vi "5_1_2.vi"() -> ()   [LabVIEW 2025, in "2022.lvlib"]
uses:
  2022.lvlib
  <vilib>/Utility/miscctls.llb/LVMapReplaceAction.ctl
panel:
  in  "Solution":bool
  out "string":string
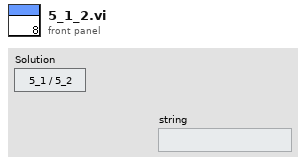
[diagram p1: front panel]
types:
  T1 = cluster{"Crane Stock":string, "Procedure":string}
  T2 = typedef "LVMapReplaceAction.ctl" = enum32{"Modify Entry only if found", "Add or Modify Entry", "Delete Entry"}
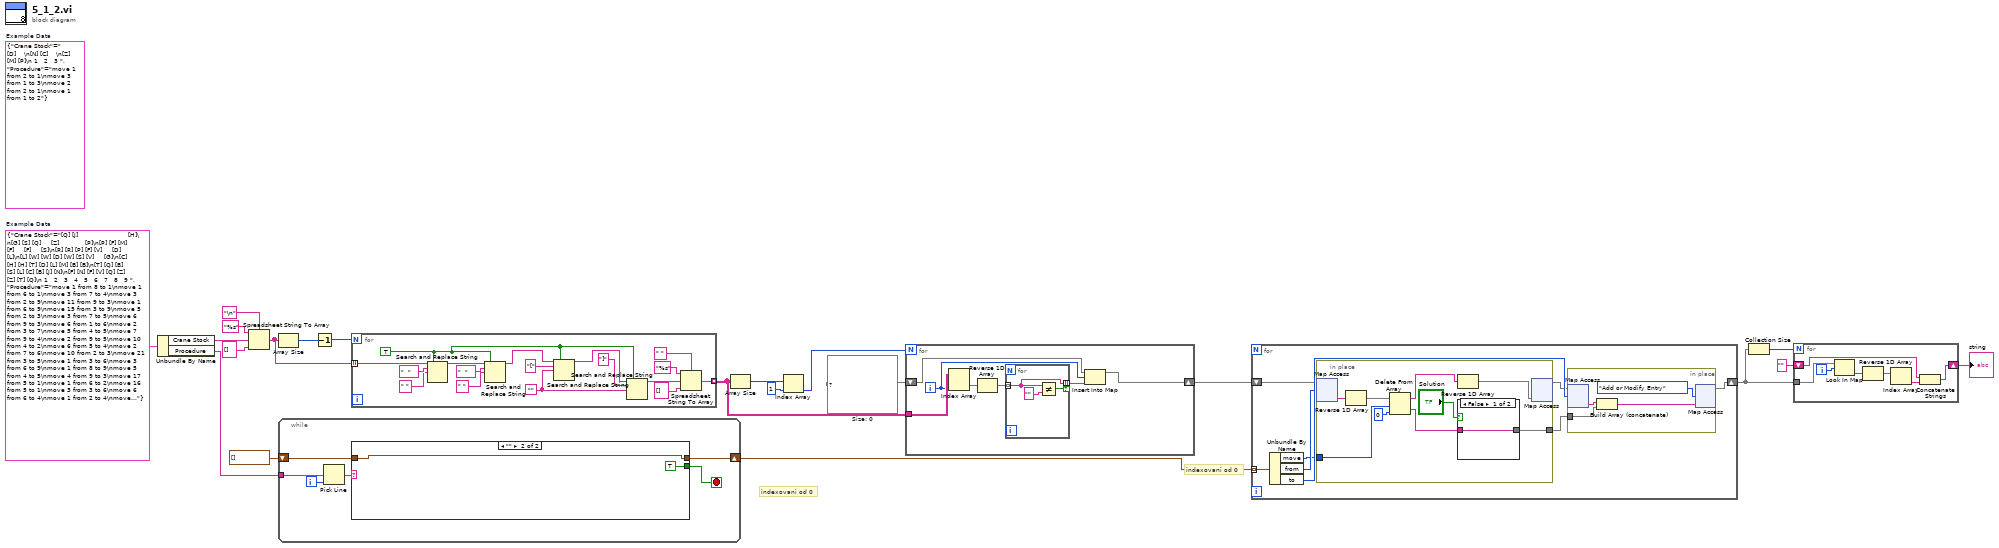
[diagram p0: block diagram]
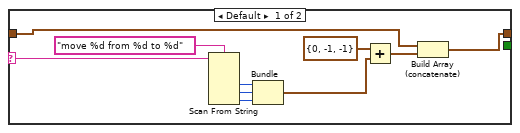
[diagram p2: hidden frame]
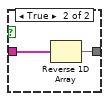
[diagram p3: hidden frame]
diagram:
  (unwired) T1 {"Crane Stock"="   [D]    \n[N] [C]    \n[Z] [M] [P]\n 1   2   3 ", "Procedure"="move 1 from 2 to 1\nmove 3 from 1 to 3\nmove 2 from 2 to 1\nmove 1 from 1 to 2"}  # Example Data
  w12 = map{i32, string[]} {}  # Size: 0
  w1 = T1 {"Crane Stock"="[Q] [J]                         [H]\n[G] [S] [Q]     [Z]             [P]\n[P] [F] [M]     [F]     [F]     [S]\n[R] [R] [P] [F] [V]     [D]     [L]\n[L] [W] [W] [D] [W] [S] [V]     [G]\n[C] [H] [H] [T] [D] [L] [M] [B] [B]\n[T] [Q] [B] [S] [L] [C] [B] [J] [N]\n[F] [N] [F] [V] [Q] [Z] [Z] [T] [Q]\n 1   2   3   4   5   6   7   8   9 ", "Procedure"="move 1 from 8 to 1\nmove 1 from 6 to 1\nmove 3 from 7 to 4\nmove 3 from 2 to 9\nmove 11 from 9 to 3\nmove 1 from 6 to 9\nmove 15 from 3 to 9\nmove 5 from 2 to 3\nmove 3 from 7 to 5\nmove 6 from 9 to 3\nmove 6 from 1 to 6\nmove 2 from 3 to 7\nmove 5 from 4 to 5\nmove 7 from 9 to 4\nmove 2 from 9 to 5\nmove 10 from 4 to 2\nmove 6 from 5 to 4\nmove 2 from 7 to 6\nmove 10 from 2 to 3\nmove 21 from 3 to 5\nmove 1 from 3 to 6\nmove 3 from 6 to 9\nmove 1 from 8 to 9\nmove 5 from 4 to 5\nmove 4 from 9 to 3\nmove 17 from 5 to 1\nmove 1 from 6 to 2\nmove 16 from 5 to 1\nmove 3 from 3 to 6\nmove 6 from 6 to 4\nmove 1 from 2 to 4\nmove 4 from 1 to 2\nmove 2 from 6 to 2\nmove 28 from 1 to 3\nmove 1 from 9 to 7\nmove 1 from 8 to 7\nmove 1 from 5 to 4\nmove 1 from 2 to 6\nmove 1 from 3 to 1\nmove 3 from 2 to 5\nmove 1 from 6 to 3\nmove 4 from 4 to 7\nmove 5 from 5 to 2\nmove 1 from 5 to 6\nmove 6 from 1 to 3\nmove 1 from 6 to 2\nmove 26 from 3 to 6\nmove 2 from 7 to 9\nmove 4 from 7 to 3\nmove 19 from 6 to 3\nmove 6 from 2 to 4\nmove 5 from 3 to 2\nmove 1 from 9 to 7\nmove 26 from 3 to 8\nmove 6 from 4 to 3\nmove 1 from 3 to 8\nmove 1 from 6 to 7\nmove 6 from 3 to 6\nmove 6 from 6 to 4\nmove 1 from 9 to 2\nmove 2 from 4 to 9\nmove 22 from 8 to 2\nmove 2 from 6 to 5\nmove 1 from 9 to 1\nmove 1 from 6 to 5\nmove 1 from 7 to 5\nmove 3 from 6 to 7\nmove 2 from 6 to 1\nmove 1 from 1 to 5\nmove 3 from 5 to 9\nmove 4 from 8 to 4\nmove 2 from 1 to 4\nmove 18 from 2 to 1\nmove 2 from 7 to 8\nmove 3 from 9 to 5\nmove 8 from 1 to 9\nmove 5 from 9 to 3\nmove 1 from 9 to 8\nmove 2 from 9 to 4\nmove 2 from 7 to 8\nmove 5 from 5 to 7\nmove 1 from 9 to 3\nmove 4 from 8 to 4\nmove 1 from 7 to 8\nmove 4 from 4 to 3\nmove 2 from 8 to 3\nmove 1 from 8 to 9\nmove 2 from 1 to 8\nmove 3 from 4 to 5\nmove 1 from 8 to 4\nmove 1 from 9 to 3\nmove 1 from 8 to 5\nmove 8 from 1 to 8\nmove 11 from 2 to 9\nmove 12 from 3 to 5\nmove 1 from 3 to 9\nmove 1 from 8 to 5\nmove 11 from 9 to 3\nmove 4 from 5 to 9\nmove 3 from 8 to 7\nmove 3 from 7 to 8\nmove 1 from 5 to 8\nmove 7 from 4 to 3\nmove 1 from 4 to 5\nmove 1 from 2 to 8\nmove 3 from 7 to 6\nmove 3 from 4 to 8\nmove 1 from 7 to 9\nmove 2 from 4 to 7\nmove 5 from 8 to 1\nmove 3 from 6 to 5\nmove 2 from 4 to 2\nmove 1 from 9 to 4\nmove 1 from 8 to 6\nmove 1 from 2 to 9\nmove 1 from 8 to 5\nmove 3 from 8 to 4\nmove 3 from 4 to 2\nmove 4 from 3 to 9\nmove 17 from 5 to 9\nmove 9 from 9 to 6\nmove 1 from 9 to 3\nmove 5 from 6 to 3\nmove 3 from 6 to 3\nmove 8 from 9 to 5\nmove 2 from 8 to 5\nmove 1 from 4 to 8\nmove 1 from 5 to 3\nmove 1 from 8 to 5\nmove 3 from 2 to 6\nmove 3 from 1 to 4\nmove 7 from 5 to 1\nmove 1 from 2 to 6\nmove 13 from 3 to 6\nmove 2 from 7 to 8\nmove 13 from 6 to 5\nmove 3 from 5 to 7\nmove 6 from 5 to 6\nmove 1 from 7 to 6\nmove 2 from 7 to 3\nmove 1 from 6 to 8\nmove 13 from 3 to 5\nmove 9 from 5 to 9\nmove 7 from 5 to 7\nmove 17 from 9 to 2\nmove 3 from 4 to 7\nmove 9 from 2 to 9\nmove 10 from 9 to 3\nmove 8 from 7 to 8\nmove 2 from 5 to 3\nmove 4 from 2 to 6\nmove 11 from 3 to 9\nmove 9 from 6 to 5\nmove 5 from 9 to 8\nmove 1 from 3 to 1\nmove 3 from 9 to 1\nmove 2 from 5 to 2\nmove 1 from 7 to 9\nmove 2 from 9 to 4\nmove 2 from 9 to 8\nmove 13 from 1 to 8\nmove 3 from 8 to 5\nmove 27 from 8 to 1\nmove 10 from 5 to 9\nmove 1 from 7 to 2\nmove 2 from 4 to 3\nmove 10 from 9 to 6\nmove 1 from 8 to 7\nmove 15 from 1 to 9\nmove 13 from 9 to 5\nmove 15 from 5 to 7\nmove 5 from 1 to 3\nmove 8 from 7 to 1\nmove 7 from 7 to 1\nmove 16 from 1 to 8\nmove 4 from 3 to 9\nmove 4 from 1 to 7\nmove 4 from 9 to 6\nmove 5 from 2 to 7\nmove 15 from 8 to 6\nmove 1 from 9 to 1\nmove 3 from 3 to 4\nmove 1 from 9 to 7\nmove 1 from 2 to 7\nmove 1 from 2 to 7\nmove 1 from 8 to 1\nmove 3 from 4 to 8\nmove 3 from 8 to 1\nmove 8 from 6 to 8\nmove 7 from 1 to 4\nmove 11 from 6 to 8\nmove 14 from 6 to 5\nmove 13 from 8 to 7\nmove 4 from 7 to 5\nmove 15 from 7 to 4\nmove 6 from 5 to 4\nmove 2 from 5 to 9\nmove 1 from 5 to 2\nmove 3 from 8 to 5\nmove 19 from 4 to 7\nmove 10 from 5 to 8\nmove 2 from 6 to 8\nmove 1 from 4 to 8\nmove 2 from 7 to 9\nmove 9 from 7 to 4\nmove 6 from 4 to 6\nmove 11 from 4 to 8\nmove 2 from 5 to 4\nmove 5 from 6 to 4\nmove 1 from 6 to 7\nmove 3 from 9 to 5\nmove 3 from 8 to 5\nmove 3 from 7 to 6\nmove 11 from 8 to 7\nmove 1 from 9 to 5\nmove 1 from 6 to 8\nmove 1 from 2 to 1\nmove 5 from 4 to 9\nmove 2 from 4 to 1\nmove 2 from 1 to 4\nmove 1 from 1 to 9\nmove 4 from 5 to 1\nmove 1 from 4 to 6\nmove 17 from 7 to 5\nmove 9 from 8 to 7\nmove 6 from 9 to 7\nmove 3 from 1 to 9\nmove 12 from 7 to 9\nmove 12 from 9 to 5\nmove 5 from 7 to 9\nmove 17 from 5 to 3\nmove 7 from 3 to 1\nmove 5 from 1 to 5\nmove 5 from 9 to 2\nmove 4 from 3 to 5\nmove 1 from 4 to 8\nmove 5 from 2 to 1\nmove 22 from 5 to 9\nmove 3 from 7 to 6\nmove 6 from 6 to 9\nmove 2 from 5 to 4\nmove 1 from 6 to 3\nmove 2 from 4 to 1\nmove 3 from 8 to 2\nmove 1 from 3 to 4\nmove 24 from 9 to 1\nmove 4 from 3 to 9\nmove 2 from 2 to 9\nmove 2 from 3 to 1\nmove 1 from 8 to 6\nmove 1 from 6 to 9\nmove 1 from 8 to 9\nmove 2 from 7 to 4\nmove 1 from 8 to 3\nmove 1 from 4 to 7\nmove 3 from 9 to 8\nmove 1 from 2 to 1\nmove 9 from 9 to 3\nmove 1 from 8 to 7\nmove 1 from 4 to 3\nmove 2 from 9 to 7\nmove 1 from 9 to 3\nmove 2 from 8 to 4\nmove 12 from 3 to 8\nmove 2 from 1 to 7\nmove 1 from 4 to 3\nmove 30 from 1 to 5\nmove 6 from 5 to 7\nmove 12 from 7 to 2\nmove 1 from 3 to 4\nmove 2 from 1 to 3\nmove 1 from 4 to 9\nmove 10 from 5 to 7\nmove 10 from 2 to 6\nmove 8 from 8 to 3\nmove 3 from 1 to 3\nmove 5 from 6 to 3\nmove 2 from 8 to 5\nmove 1 from 9 to 2\nmove 2 from 8 to 6\nmove 4 from 7 to 2\nmove 3 from 2 to 7\nmove 2 from 7 to 5\nmove 1 from 4 to 9\nmove 11 from 3 to 1\nmove 7 from 6 to 9\nmove 3 from 2 to 3\nmove 10 from 1 to 7\nmove 14 from 7 to 5\nmove 3 from 7 to 6\nmove 5 from 9 to 7\nmove 29 from 5 to 7\nmove 6 from 3 to 9\nmove 2 from 9 to 7\nmove 15 from 7 to 5\nmove 11 from 5 to 6\nmove 5 from 9 to 5\nmove 10 from 5 to 8\nmove 1 from 2 to 4\nmove 1 from 8 to 2\nmove 2 from 4 to 3\nmove 2 from 5 to 9\nmove 8 from 8 to 9\nmove 11 from 9 to 3\nmove 1 from 1 to 8\nmove 18 from 7 to 3\nmove 1 from 9 to 3\nmove 28 from 3 to 5\nmove 12 from 6 to 7\nmove 1 from 2 to 9\nmove 15 from 7 to 2\nmove 1 from 8 to 1\nmove 10 from 2 to 9\nmove 10 from 5 to 3\nmove 2 from 2 to 3\nmove 18 from 3 to 4\nmove 6 from 9 to 4\nmove 1 from 1 to 7\nmove 1 from 6 to 4\nmove 1 from 8 to 2\nmove 1 from 9 to 4\nmove 2 from 9 to 4\nmove 19 from 4 to 3\nmove 1 from 7 to 9\nmove 1 from 9 to 7\nmove 1 from 6 to 8\nmove 3 from 2 to 8\nmove 2 from 9 to 5\nmove 15 from 3 to 1\nmove 7 from 5 to 1\nmove 3 from 4 to 9\nmove 1 from 7 to 2\nmove 3 from 3 to 1\nmove 6 from 5 to 2\nmove 3 from 3 to 9\nmove 4 from 9 to 2\nmove 5 from 5 to 3\nmove 1 from 3 to 5\nmove 3 from 5 to 7\nmove 3 from 8 to 5\nmove 1 from 7 to 5\nmove 4 from 5 to 1\nmove 4 from 4 to 2\nmove 2 from 7 to 8\nmove 12 from 1 to 6\nmove 1 from 8 to 6\nmove 6 from 2 to 3\nmove 9 from 3 to 8\nmove 1 from 3 to 4\nmove 3 from 6 to 1\nmove 2 from 9 to 2\nmove 1 from 4 to 5\nmove 2 from 8 to 3\nmove 10 from 2 to 1\nmove 2 from 4 to 7\nmove 12 from 1 to 4\nmove 1 from 5 to 1\nmove 7 from 4 to 9\nmove 2 from 3 to 2\nmove 6 from 9 to 2\nmove 1 from 9 to 1\nmove 1 from 7 to 8\nmove 5 from 6 to 7\nmove 3 from 6 to 1\nmove 6 from 2 to 3\nmove 2 from 4 to 3\nmove 1 from 6 to 8\nmove 1 from 6 to 7\nmove 8 from 3 to 9\nmove 2 from 4 to 5\nmove 3 from 2 to 4\nmove 10 from 8 to 2\nmove 22 from 1 to 9\nmove 9 from 2 to 4\nmove 1 from 1 to 3\nmove 1 from 3 to 2\nmove 3 from 2 to 4\nmove 2 from 7 to 1\nmove 14 from 4 to 2\nmove 2 from 1 to 8\nmove 2 from 4 to 5\nmove 4 from 7 to 8\nmove 24 from 9 to 6\nmove 3 from 5 to 9\nmove 1 from 9 to 8\nmove 1 from 5 to 2\nmove 1 from 6 to 7\nmove 6 from 9 to 1\nmove 1 from 7 to 3\nmove 5 from 8 to 6\nmove 9 from 6 to 3\nmove 4 from 1 to 4\nmove 2 from 1 to 2\nmove 11 from 6 to 3\nmove 13 from 3 to 2\nmove 2 from 9 to 8\nmove 8 from 3 to 8\nmove 2 from 8 to 5\nmove 1 from 7 to 5\nmove 3 from 6 to 3\nmove 11 from 8 to 5\nmove 13 from 2 to 4\nmove 10 from 5 to 2\nmove 2 from 3 to 4\nmove 2 from 5 to 7\nmove 15 from 4 to 9\nmove 2 from 7 to 4\nmove 2 from 4 to 2\nmove 2 from 4 to 9\nmove 2 from 4 to 2\nmove 1 from 3 to 8\nmove 1 from 8 to 1\nmove 1 from 1 to 2\nmove 1 from 6 to 3\nmove 7 from 2 to 4\nmove 1 from 5 to 3\nmove 7 from 9 to 1\nmove 7 from 1 to 2\nmove 4 from 6 to 9\nmove 12 from 9 to 7\nmove 6 from 7 to 5\nmove 1 from 3 to 5\nmove 7 from 4 to 7\nmove 3 from 7 to 8\nmove 3 from 8 to 6\nmove 18 from 2 to 9\nmove 7 from 2 to 3\nmove 15 from 9 to 4\nmove 3 from 3 to 9\nmove 1 from 3 to 1\nmove 3 from 5 to 4\nmove 1 from 1 to 2\nmove 1 from 9 to 2\nmove 2 from 6 to 2\nmove 5 from 7 to 6\nmove 5 from 2 to 7\nmove 3 from 3 to 4\nmove 5 from 5 to 3\nmove 6 from 7 to 4\nmove 9 from 4 to 2\nmove 18 from 4 to 9\nmove 6 from 2 to 1\nmove 1 from 1 to 9\nmove 4 from 7 to 4\nmove 7 from 2 to 4\nmove 1 from 2 to 8\nmove 1 from 4 to 2\nmove 4 from 3 to 4\nmove 16 from 9 to 5\nmove 9 from 9 to 8\nmove 1 from 9 to 7\nmove 4 from 1 to 2\nmove 2 from 5 to 4\nmove 10 from 5 to 4\nmove 4 from 2 to 1\nmove 5 from 1 to 2\nmove 1 from 8 to 5\nmove 1 from 6 to 5\nmove 4 from 8 to 5\nmove 2 from 6 to 9\nmove 3 from 6 to 2\nmove 2 from 9 to 1\nmove 1 from 7 to 6\nmove 1 from 3 to 8\nmove 9 from 5 to 9\nmove 4 from 8 to 1\nmove 2 from 8 to 2\nmove 1 from 5 to 7\nmove 9 from 9 to 8\nmove 1 from 7 to 5\nmove 9 from 8 to 2\nmove 6 from 1 to 6\nmove 6 from 2 to 6\nmove 10 from 2 to 5\nmove 5 from 2 to 1\nmove 1 from 3 to 5\nmove 8 from 5 to 4\nmove 5 from 1 to 3\nmove 10 from 6 to 8\nmove 3 from 6 to 9\nmove 4 from 3 to 1\nmove 5 from 8 to 2\nmove 4 from 5 to 9\nmove 1 from 3 to 7\nmove 1 from 7 to 3\nmove 1 from 8 to 6\nmove 1 from 6 to 1\nmove 15 from 4 to 8\nmove 5 from 9 to 2\nmove 1 from 9 to 1\nmove 1 from 1 to 3\nmove 6 from 4 to 8\nmove 12 from 8 to 7\nmove 1 from 3 to 5\nmove 3 from 1 to 9\nmove 13 from 4 to 9\nmove 5 from 7 to 2\nmove 1 from 5 to 4\nmove 8 from 9 to 5\nmove 6 from 2 to 5\nmove 2 from 5 to 6"}  # Example Data
  # "indexovani od 0"
  # "indexovani od 0"
  n1 = Unbundle By Name(w1) -> ("Crane Stock"=w15:string, "Procedure"=w13:string)
  n2 = Spreadsheet String To Array(delimiter (Tab)="\n", format string="%s", spreadsheet string=w15, array type (2D Dbl)=string[] []) -> (array=w18:string[])
  n3 = Array Size(array=w18) -> (size(s)=w17:i32)
  n4 = while {
    tunnel: w13 -> [w27]
    shift-right: [w23] -> w10
    shift-left: cluster{"move":i32, "from":i32, "to":i32}[] [] -> [w22]
    i -> [w26]
    stop <- w24 stop-if-true
    n5 = Pick Line(multi-line string=w27, line index=w26) -> (output string=w25:string)  [unwired: 1 in]
    n6 = case shown="\"\"" w25 {
      selector: w25 -> [w37 _]
      tunnel: [_ TRUE] -> w24
      tunnel: [w32 w38] -> w23
      tunnel: w22 -> [w31 w38]
      frame Default {
        n7 = Scan From String(format string="move %d from %d to %d", input string=w37) -> (output 1=w35:i32, output 2=w34:i32, output 3=w33:i32)  [unwired: 5 in, 3 out]
        n8 = Bundle(w35, w34, w33) -> (w29:cluster{i32, i32, i32})  [unwired: 1 in]
        n9 = Add(x=cluster{"move":i32, "from":i32, "to":i32} {"move"=0, "from"=-1, "to"=-1}, y=w29) -> (x+y=w28:cluster{i32, i32, i32})
        n10 = Build Array (concatenate)(w31, w28) -> (w32:cluster{"move":i32, "from":i32, "to":i32}[])
      }
      frame "" {
      }
    }
  }
  n11 = Decrement(x=w17) -> (x-1=w16:i32)
  n12 = for {
    N: w16 -> [_]
    tunnel: w18 -> [w48] mode=indexing
    tunnel: [w40] -> w5 mode=indexing
    w41 = TRUE ("replace all? (F)")
    w49 = ""
    n13 = Search and Replace String(replace all?=w41, input string=w48, search string="  " ("delimiter (Tab)"), replace string=" " ("delimiter (Tab)")) -> (result string=w43:string)  [unwired: 4 in, 3 out]
    n14 = Search and Replace String(replace all?=w41, input string=w43, search string="  " ("delimiter (Tab)"), replace string=" " ("delimiter (Tab)")) -> (result string=w42:string)  [unwired: 4 in, 3 out]
    n15 = Search and Replace String(replace all?=w41, input string=w42, search string="[" ("input string"), replace string=w49) -> (result string=w53:string)  [unwired: 4 in, 3 out]
    n16 = Search and Replace String(replace all?=w41, input string=w53, search string="]", replace string=w49) -> (result string=w50:string)  [unwired: 4 in, 3 out]
    n17 = Spreadsheet String To Array(delimiter (Tab)=" ", format string="%s", spreadsheet string=w50, array type (2D Dbl)=string[] []) -> (array=w40:string[])
  }
  n18 = Array Size(array=w5) -> (size(s)=w4:i32[])
  n19 = Index Array(array=w4, index=1) -> (element=w2:i32)
  n20 = for {
    N: w2 -> [_]
    tunnel: w5 -> [w61]
    shift-right: [w62] -> w11
    shift-left: w12 -> [w63]
    i -> [w59]
    n21 = Index Array(array=w61, index (col)=w59) -> (element=w60:string[])  [unwired: 1 in]
    n22 = Reverse 1D Array(array=w60) -> (reversed array=w58:string[])
    n23 = for {
      tunnel: w58 -> [w65] mode=indexing
      tunnel: [w65] -> w57 mode=indexing if=w64
      n24 = Not Equal?(x=w65, y="") -> (x != y?=w64:bool)
    }
    n25 = Insert Into Map(map in=w63, key=w59, value=w57) -> (map out=w62:map{i32, string[]})  [unwired: 2 out]
  }
  n26 = for {
    tunnel: w10 -> [w74] mode=indexing
    shift-right: [w72] -> w8
    shift-left: w11 -> [w71]
    n27 = Unbundle By Name(w74) -> ("move"=w67:i32, "from"=w69:i32, "to"=w73:i32)
    n28 = in-place {
      in-place-border: [w75] -> w68
      in-place-border: w67 -> [w81]
      n29 = in-place-map #1(w71, w69) -> (w80:string[])  [unwired: 1 in, 1 out]
      n30 = Reverse 1D Array(array=w80) -> (reversed array=w78:string[])
      n31 = Delete From Array(array=w78, length=w81, index=0) -> (deleted portion=w77:string[], array with subset deleted=w82:string[])
      n32 = Reverse 1D Array(array=w82) -> (reversed array=w79:string[])
      n33 = case shown="False" "Solution" {
        tunnel: w77 -> [w84 w86]
        tunnel: [w84 w85] -> w75
        frame False {
        }
        frame True {
          n34 = Reverse 1D Array(array=w86) -> (reversed array=w85:string[])
        }
      }
      n35 = in-place-map #1(w79) -> (w70:map{i32, string[]})  [unwired: 1 in, 2 out]
    }
    n36 = in-place {
      in-place-border: w68 -> [w88]
      n37 = in-place-map #2(w70, w73) -> (w87:string[])  [unwired: 1 in, 1 out]
      n38 = Build Array (concatenate)(w87, w88) -> (w89:string[])
      n39 = in-place-map #2(w89, LVMapReplaceAction."Add or Modify Entry" ("action")) -> (w72:map{i32, string[]})  [unwired: 2 out]
    }
  }
  n40 = Collection Size(1:w8) -> (0:w9:i32)
  n41 = for {
    N: w9 -> [_]
    tunnel: w8 -> [w94]
    shift-right: [w92] -> w6
    shift-left: "" ("string") -> [w93]
    i -> [w97]
    n42 = Look In Map(map=w94, key=w97) -> (value=w96:string[])  [unwired: 1 in, 1 out]
    n43 = Reverse 1D Array(array=w96) -> (reversed array=w95:string[])
    n44 = Index Array(array=w95) -> (element=w91:string)  [unwired: 1 in]
    n45 = Concatenate Strings(w93, w91) -> (w92:string)
  }
  "string" <- w6
